vi "GA Get Stop Dec.vi"(8 "error in (no error)":errorcluster caption="错误输入（无错误）", 9 "pDecAbruptStop":dbl, 10 "pDecSmoothStop":dbl, 11 "nAxisNum":i16) -> (0 "error out":errorcluster caption="错误输出", 1 "pDecAbruptStop out":dbl, 2 "pDecSmoothStop out":dbl, 3 "function return":i32)   [LabVIEW 2015, in "GAS.lvlib"]
doc: "extern \"C\" __declspec(dllimport) int GA_GetStopDec(short nAxisNum,double *pDecSmoothStop,double *pDecAbruptStop);"
uses:
  <userlib>/BP_GAS/GAS.lvlib
  <userlib>/BP_GAS/GAS.dll
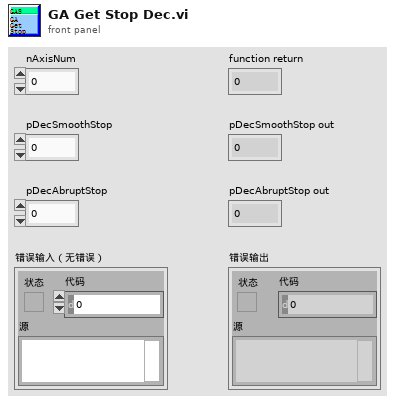
[diagram p1: front panel]
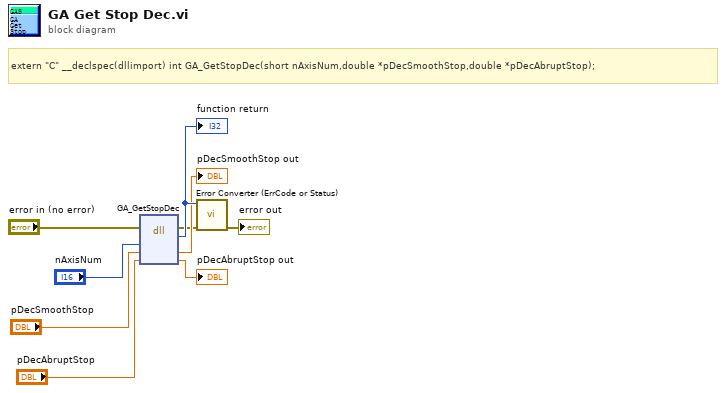
[diagram p0: block diagram]
diagram:
  # "extern \"C\" __declspec(dllimport) int GA_GetStopDec(short nAxisNum,double *pDecSmoothStop,double *pDecAbruptStop);"
  n1 = dll-call lib="E:/Program Files (x86)/National Instruments/LabVIEW 2015/user.lib/BP_GAS/GAS.*" fn="GA_GetStopDec"(error in="error in (no error)", "nAxisNum"="nAxisNum", "pDecSmoothStop"="pDecSmoothStop", "pDecAbruptStop"="pDecAbruptStop") -> (error out=w2:errorcluster, w9:i32, "pDecSmoothStop"=→"pDecSmoothStop out":dbl, "pDecAbruptStop"=→"pDecAbruptStop out":dbl)  [unwired: 3 in, 1 out]
  "function return" <- w9
  n2 = call "Error Converter (ErrCode or Status).vi"("error in (no error)"=w2, "error code"=w9) -> ("error out"=→"error out":errorcluster)  [unwired: 9 in]
